vi "Example One Stage_Patrick.vi"() -> ()   [LabVIEW 2019]
uses:
  Class/Controller/Controller.lvclass
  <vilib>/Platform/TimedLoop/XDataNode/timing_clust.ctl
  <vilib>/Platform/TimedLoop/XDataNode/nitl_modes.ctl
  <vilib>/Platform/TimedLoop/XDataNode/wakeup.ctl
  <vilib>/platform/TimedLoop/XDataNode/XDataNode.xnode
  <vilib>/Platform/TimedLoop/XDataNode/XDNodeRunTimeDep.lvlib
panel:
  out "Desired Position\n[selected units]":dbl
  out "Encoder position \n[selected units]":dbl
  in  "Tab Control":enum32{"Motion", "Settings"}(tab)
  in  "Zero Output":bool
  in  "Go to Home":bool
  in  "Scan Right":bool
  in  "Scan Left":bool
  in  "Continue":bool
  in  "Stop":bool
  in  "Make Step Right":bool
  in  "Step Size \n[selected units]":dbl=1.0 format="%#.2f"
  in  "Make Step Left":bool
  in  "Desired Speed \n[1µm/s or 0,01deg /s]":dbl=10000.0 format="%#.2f"
  in  "Desired Position \n[selected units]":dbl format="%#.2f"
  in  "Find Index":bool
  in  "Reset":bool
  out "error out":errorcluster
  in  "Working Units":string(combo)="1000000,0"
  out "StatusBits":T1
  out "Status Info":T2
  in  "Axis Resolution":string(combo)="3.49065850399"
  in  "Axis Letter":string="X"
  in  "Baudrate":dbl=9600.0
  in  "COM Port":refnum<visa-resource-name>="COM4"
  in  "Controller.lvclass":refnum<class "Controller.lvclass">
  out "Waveform Chart":dbl(graph)=-0.078
  in  "STOP PROGRAM":bool
  # "Visualization"
  # "Extra information"
  # "READ ME FIRST"
  # "Configuration"
  # "Stage 1"
  # "Driver 1"
  # "Stage 1"
  # "How to run:"
  # "BEFORE RUNNING:"
  # "1, Select COM Port"
  # "2. Select baudrate"
  # "3. For each axis:"
  # "3.1 Specify correct axis name (1 letter)"
  # "3.2 Specify correct resolution"
  # "4. Run VI"
  # "WHEN RUNNING, YOU HAVE TO FIRST PUSH \"FIND INDEX\" FOR EACH STAGE.\nThe stages will start moving and find its position. After that you can control the stages"
  # "NOTES: Do this only the first time"
  # "1. Replace the settings_default.txt file with\nthe file we provided on a USB stick."
  # "2.    Make sure there are no comments in the\nsettings_default.txt file. ONLY lines like: \"X:DPOS=100\" so NO \"%\" in front or at the end of the line."
  # "Position Information"
  # "STOP BUTTON"
  # "3.  In your settings_default.txt file:\nEvery line that contains SSPD or MSPD: multiply that value with:\n - 1000 for a lineair stage \n - 100 for a rotating stage"
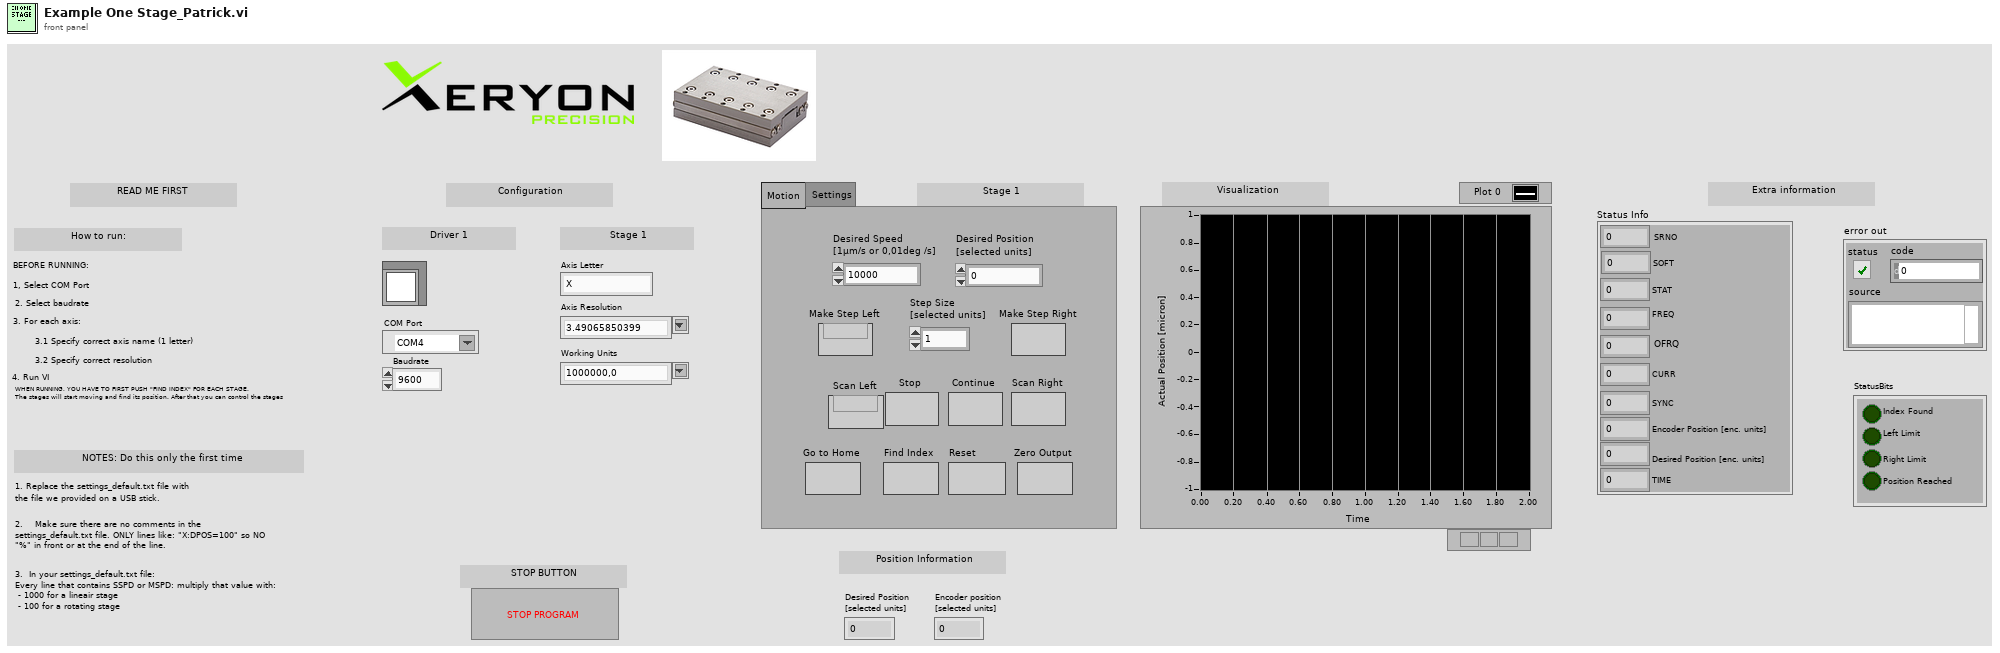
[diagram p1: front panel]
types:
  T1 = cluster{"Index Found":bool, "Left Limit":bool, "Right Limit":bool, "Position Reached":bool}
  T2 = cluster{"SRNO":dbl, "SOFT":dbl, "STAT":dbl, "FREQ":dbl, "OFRQ":dbl, "CURR":dbl, "SYNC":dbl, "Encoder Position [enc. units]":dbl, "Desired Position [enc. units]":dbl, "TIME":dbl}
  T3 = typedef "XDNodeRunTimeDep.lvlib/timing_clust.ctl" = cluster{"Expected End [f-1]":u64, "Actual End [f-1]":u64, "Finished Late? [f-1]":bool, "Expected End [i-1]":u64, "Actual End [i-1]":u64, "Finished Late? [i-1]":bool, "Expected Start [i]":u64, "Actual Start [i]":u64, "Expected Start [f]":u64, "Actual Start [f]":u64, "Source Name":string, "Structure Name":string, "Period":i64, "Deadline":i64, "Offset":i64, "Start":i64, "Priority":i32, "Timeout":i32, "Mode":T4, "Wakeup Reason":T5, "Error":errorcluster, "Source Type":string, "Secondary Source Type":string, "Global End Time":u64, "Global Start Time":u64, "Frame Duration":u64, "Iteration Duration":u64, "Assigned CPU":i32, "I/O Scan Engine Mode":u32}
  T4 = typedef "XDNodeRunTimeDep.lvlib/nitl_modes.ctl" = enum32{"No Change", "Process missed periods, maintain original phase", "Discard missed periods, maintain original phase", "Process missed periods, ignore original phase", "Discard missed periods, ignore original phase"}
  T5 = typedef "XDNodeRunTimeDep.lvlib/wakeup.ctl" = enum32{"Normal", "Aborted", "Asynchronous wakeup", "Timing source error", "Timed loop error", "Timeout"}
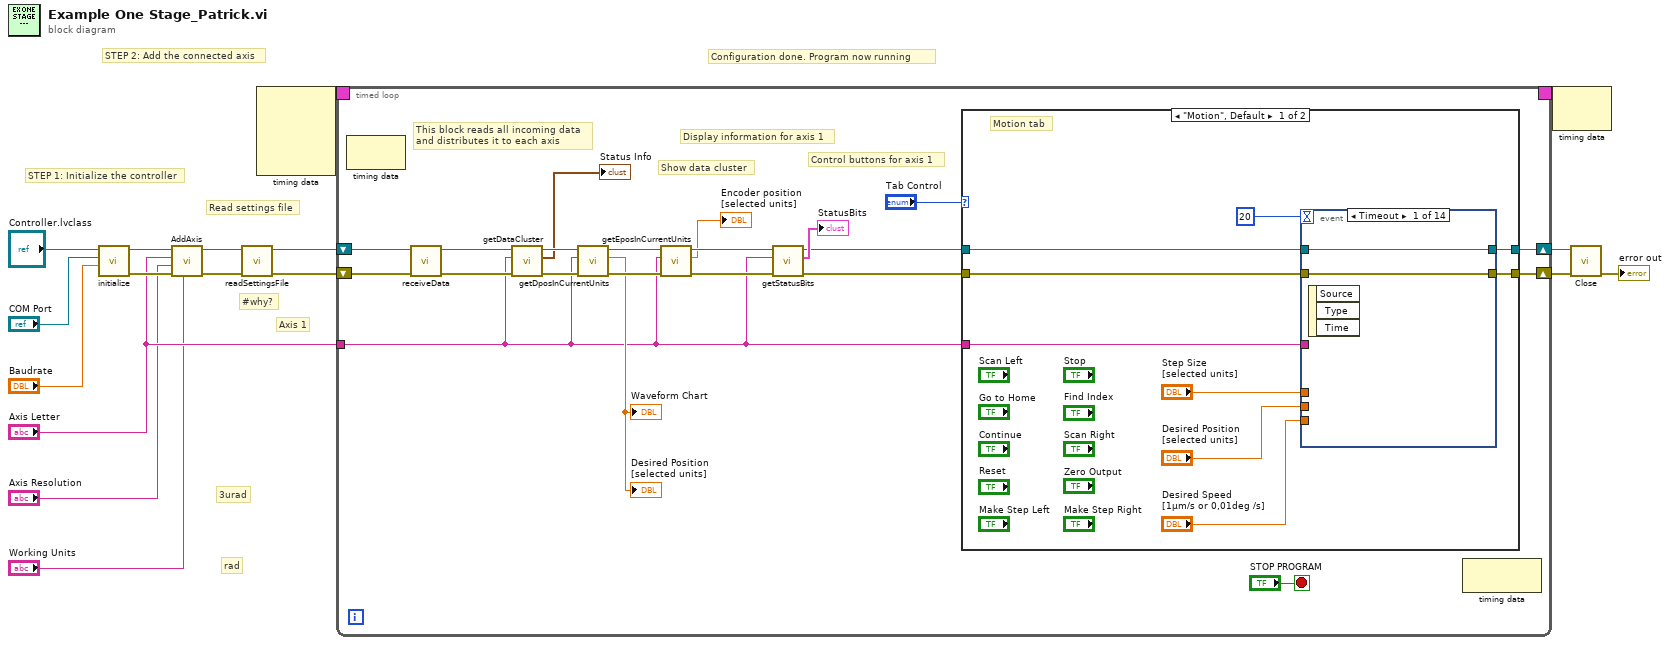
[diagram p0: block diagram]
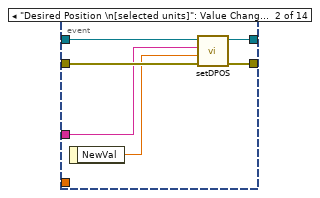
[diagram p2: hidden frame]
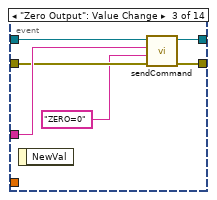
[diagram p3: hidden frame]
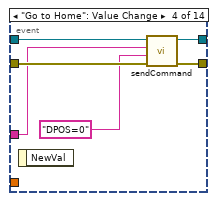
[diagram p4: hidden frame]
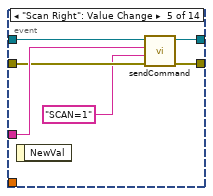
[diagram p5: hidden frame]
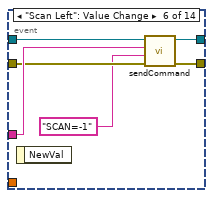
[diagram p6: hidden frame]
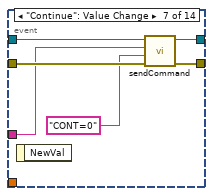
[diagram p7: hidden frame]
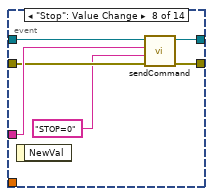
[diagram p8: hidden frame]
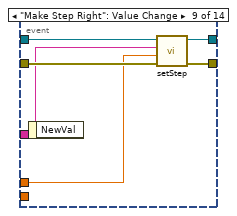
[diagram p9: hidden frame]
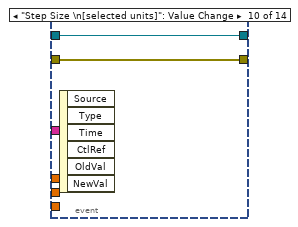
[diagram p10: hidden frame]
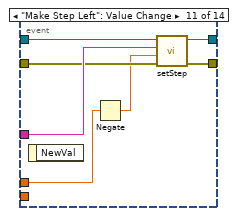
[diagram p11: hidden frame]
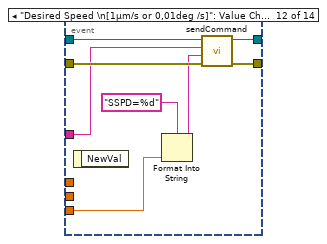
[diagram p12: hidden frame]
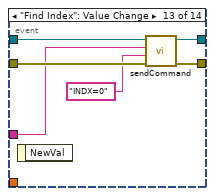
[diagram p13: hidden frame]
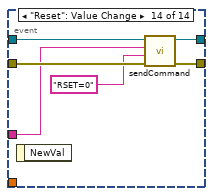
[diagram p14: hidden frame]
diagram:
  # "rad"
  # "3urad"
  # "#why?"
  # "Axis 1"
  # "Configuration done. Program now running"
  # "Read settings file"
  # "STEP 2: Add the connected axis"
  # "STEP 1: Initialize the controller"
  n1 = call-dynamic "initialize.vi"("Baudrate"="Baudrate", "COM Port"="COM Port", "Controller in"="Controller.lvclass") -> ("error out"=w16:errorcluster, "Controller out"=w17:refnum<class "Controller.lvclass">)  [unwired: 7 in]
  n2 = call-dynamic "AddAxis.vi"("Units"="Working Units", "error in (no error)"=w16, "Encoder Resolution"="Axis Resolution", "Axis Letter"="Axis Letter", "Controller in"=w17) -> ("error out"=w11:errorcluster, "Controller out"=w12:refnum<class "Controller.lvclass">)  [unwired: 5 in]
  n3 = call-dynamic "readSettingsFile.vi"("error in (no error)"=w11, "Controller in"=w12) -> ("error out"=w13:errorcluster, "Controller out"=w14:refnum<class "Controller.lvclass">)  [unwired: 8 in]
  n4 = node-c288() -> (w8:T3)  [unwired: 4 in]
  n5 = timed-loop {
    shift-right: [w19] -> w3
    shift-left: w14 -> [w38]
    tunnel: "Axis Letter" -> [w21]
    shift-right: [w18] -> w2
    shift-left: w13 -> [w27]
    timing: w8 -> [_]
    timing-out: [_] -> w7
    stop <- "STOP PROGRAM" stop-if-true
    # "Control buttons for axis 1"
    # "Display information for axis 1"
    # "Show data cluster"
    # "This block reads all incoming data\nand distributes it to each axis"
    n6 = node-c288() -> ()  [unwired: 1 in, 1 out]
    n7 = call-dynamic "receiveData.vi"("error in (no error)"=w27, "Controller in"=w38) -> ("error out"=w36:errorcluster, "Controller out"=w37:refnum<class "Controller.lvclass">)  [unwired: 8 in]
    n8 = call-dynamic "getDataCluster.vi"("error in (no error)"=w36, "Axis Letter"=w21, "Controller in"=w37) -> ("error out"=w31:errorcluster, "Information"=→"Status Info":T2, "Controller out"=w34:refnum<class "Controller.lvclass">)  [unwired: 6 in]
    n9 = call-dynamic "getDposInCurrentUnits.vi"("error in (no error)"=w31, "Axis Letter"=w21, "Controller in"=w34) -> ("error out"=w30:errorcluster, "DPOS In Current Units"=→"Waveform Chart" →"Desired Position\n[selected units]":dbl, "Controller out"=w33:refnum<class "Controller.lvclass">)  [unwired: 6 in]
    n10 = call-dynamic "getEposInCurrentUnits.vi"("error in (no error)"=w30, "Axis Letter"=w21, "Controller in"=w33) -> ("error out"=w29:errorcluster, "EPOS In Current Units"=→"Encoder position \n[selected units]":dbl, "Controller out"=w32:refnum<class "Controller.lvclass">)  [unwired: 6 in]
    n11 = call-dynamic "getStatusBits.vi"("error in (no error)"=w29, "Axis Letter"=w21, "Controller in"=w32) -> ("error out"=w24:errorcluster, "StatusBits"=→"StatusBits":T1, "Controller out"=w20:refnum<class "Controller.lvclass">)  [unwired: 6 in]
    n12 = case shown="\"Motion\", Default" "Tab Control" {
      tunnel: w20 -> [w49 w130]
      tunnel: w24 -> [w48 w129]
      tunnel: [w47 w130] -> w19
      tunnel: [w46 w129] -> w18
      tunnel: w21 -> [w44 _]
      frame "Motion", Default {
        # "Motion tab"
        n13 = event shown="[0] Timeout" {
          selector: _ -> [_ _ _ _ _ _ _ _ _ _ _ _ _ _]
          dyn-events: _ -> [_ _ _ _ _ _ _ _ _ _ _ _ _ _]
          timeout: 20 -> [_ _ _ _ _ _ _ _ _ _ _ _ _ _]
          tunnel: w49 -> [w51 w57 w63 w69 w75 w81 w87 w93 w98 w101 w108 w116 w122 w128]
          tunnel: w48 -> [w50 w56 w61 w68 w73 w79 w86 w91 w99 w100 w106 w115 w121 w127]
          tunnel: [w51 w54 w59 w66 w71 w77 w84 w89 w96 w101 w104 w113 w119 w126] -> w47
          tunnel: [w50 w55 w60 w67 w72 w78 w85 w90 w95 w100 w105 w114 w120 w125] -> w46
          tunnel: w44 -> [_ w52 w62 w65 w74 w80 w83 w92 w97 _ w107 w112 w118 w124]
          tunnel: "Step Size \n[selected units]" -> [_ _ _ _ _ _ _ _ w94 _ w103 _ _ _]
          tunnel: "Desired Position \n[selected units]" -> [_ _ _ _ _ _ _ _ _ _ _ _ _ _]
          tunnel: "Desired Speed \n[1µm/s or 0,01deg /s]" -> [_ _ _ _ _ _ _ _ _ _ _ w109 _ _]
          event Timeout {
            n14 = event-data() -> ()  [unwired: 1 in, 3 out]
          }
          event "Desired Position \n[selected units]": Value Change {
            n15 = event-data() -> ("NewVal"=w53:dbl)  [unwired: 1 in]
            n16 = call-dynamic "setDPOS.vi"("error in (no error)"=w56, "DPOS In Current Units"=w53, "Axis Letter"=w52, "Controller in"=w57) -> ("error out"=w55:errorcluster, "Controller out"=w54:refnum<class "Controller.lvclass">)  [unwired: 6 in]
          }
          event "Zero Output": Value Change {
            n17 = event-data() -> ()  [unwired: 1 in, 1 out]
            n18 = call-dynamic "sendCommand.vi"("error in (no error)"=w61, "Command"="ZERO=0", "Axis Letter"=w62, "Controller in"=w63) -> ("error out"=w60:errorcluster, "Controller out"=w59:refnum<class "Controller.lvclass">)  [unwired: 6 in]
          }
          event "Go to Home": Value Change {
            n19 = event-data() -> ()  [unwired: 1 in, 1 out]
            n20 = call-dynamic "sendCommand.vi"("error in (no error)"=w68, "Command"="DPOS=0", "Axis Letter"=w65, "Controller in"=w69) -> ("error out"=w67:errorcluster, "Controller out"=w66:refnum<class "Controller.lvclass">)  [unwired: 6 in]
          }
          event "Scan Right": Value Change {
            n21 = event-data() -> ()  [unwired: 1 in, 1 out]
            n22 = call-dynamic "sendCommand.vi"("error in (no error)"=w73, "Command"="SCAN=1", "Axis Letter"=w74, "Controller in"=w75) -> ("error out"=w72:errorcluster, "Controller out"=w71:refnum<class "Controller.lvclass">)  [unwired: 6 in]
          }
          event "Scan Left": Value Change {
            n23 = event-data() -> ()  [unwired: 1 in, 1 out]
            n24 = call-dynamic "sendCommand.vi"("error in (no error)"=w79, "Command"="SCAN=-1", "Axis Letter"=w80, "Controller in"=w81) -> ("error out"=w78:errorcluster, "Controller out"=w77:refnum<class "Controller.lvclass">)  [unwired: 6 in]
          }
          event "Continue": Value Change {
            n25 = event-data() -> ()  [unwired: 1 in, 1 out]
            n26 = call-dynamic "sendCommand.vi"("error in (no error)"=w86, "Command"="CONT=0", "Axis Letter"=w83, "Controller in"=w87) -> ("error out"=w85:errorcluster, "Controller out"=w84:refnum<class "Controller.lvclass">)  [unwired: 6 in]
          }
          event "Stop": Value Change {
            n27 = event-data() -> ()  [unwired: 1 in, 1 out]
            n28 = call-dynamic "sendCommand.vi"("error in (no error)"=w91, "Command"="STOP=0", "Axis Letter"=w92, "Controller in"=w93) -> ("error out"=w90:errorcluster, "Controller out"=w89:refnum<class "Controller.lvclass">)  [unwired: 6 in]
          }
          event "Make Step Right": Value Change {
            n29 = event-data() -> ()  [unwired: 1 in, 1 out]
            n30 = call-dynamic "setStep.vi"("error in (no error)"=w99, "Step Value"=w94, "Axis Letter"=w97, "Controller in"=w98) -> ("error out"=w95:errorcluster, "Controller out"=w96:refnum<class "Controller.lvclass">)  [unwired: 6 in]
          }
          event "Step Size \n[selected units]": Value Change {
            n31 = event-data() -> ()  [unwired: 1 in, 6 out]
          }
          event "Make Step Left": Value Change {
            n32 = event-data() -> ()  [unwired: 1 in, 1 out]
            n33 = Negate(x=w103) -> (-x=w102:dbl)
            n34 = call-dynamic "setStep.vi"("error in (no error)"=w106, "Step Value"=w102, "Axis Letter"=w107, "Controller in"=w108) -> ("error out"=w105:errorcluster, "Controller out"=w104:refnum<class "Controller.lvclass">)  [unwired: 6 in]
          }
          event "Desired Speed \n[1µm/s or 0,01deg /s]": Value Change {
            n35 = event-data() -> ()  [unwired: 1 in, 1 out]
            n36 = Format Into String(format string="SSPD=%d", w109) -> (resulting string=w111:string)  [unwired: 2 in, 1 out]
            n37 = call-dynamic "sendCommand.vi"("error in (no error)"=w115, "Command"=w111, "Axis Letter"=w112, "Controller in"=w116) -> ("error out"=w114:errorcluster, "Controller out"=w113:refnum<class "Controller.lvclass">)  [unwired: 6 in]
          }
          event "Find Index": Value Change {
            n38 = event-data() -> ()  [unwired: 1 in, 1 out]
            n39 = call-dynamic "sendCommand.vi"("error in (no error)"=w121, "Command"="INDX=0", "Axis Letter"=w118, "Controller in"=w122) -> ("error out"=w120:errorcluster, "Controller out"=w119:refnum<class "Controller.lvclass">)  [unwired: 6 in]
          }
          event "Reset": Value Change {
            n40 = event-data() -> ()  [unwired: 1 in, 1 out]
            n41 = call-dynamic "sendCommand.vi"("error in (no error)"=w127, "Command"="RSET=0", "Axis Letter"=w124, "Controller in"=w128) -> ("error out"=w125:errorcluster, "Controller out"=w126:refnum<class "Controller.lvclass">)  [unwired: 6 in]
          }
        }
      }
      frame "Settings" {
      }
    }
    n42 = node-c288() -> ()  [unwired: 1 in, 1 out]
  }
  n43 = node-c288(w7) -> ()  [unwired: 1 out]
  n44 = call-dynamic "Close.vi"("error in (no error)"=w2, "Controller in"=w3) -> ("error out"=→"error out":errorcluster)  [unwired: 8 in, 1 out]
